vi "1.2.vi"() -> ()   [LabVIEW 2020]
panel:
  in  "Knob":dbl(knob) scale=0.0..10.0
  out "Meter":dbl(knob) scale=0.0..10.0
  out "Boolean 2":bool
  in  "Boolean":bool
  out "Numeric 2":i64
  in  "Numeric":i64
  out "String 2":string
  in  "String":string
  # "Tipo String"
  # "Tipo INT"
  # "Tipo Boolean"
  # "Tipo DBL"
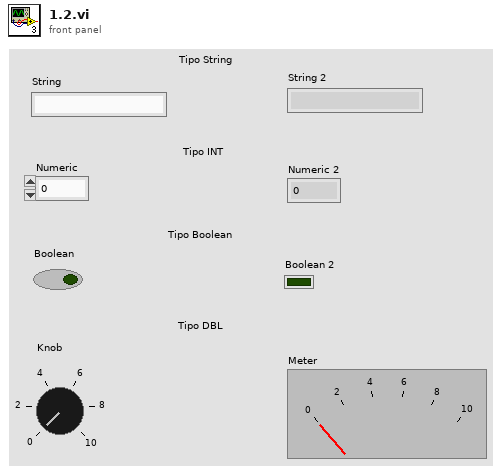
[diagram p1: front panel]
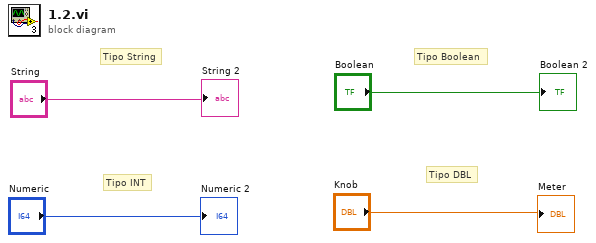
[diagram p0: block diagram]
diagram:
  # "Tipo DBL"
  # "Tipo Boolean"
  # "Tipo INT"
  # "Tipo String"
  "String 2" <- "String"
  "Numeric 2" <- "Numeric"
  "Boolean 2" <- "Boolean"
  "Meter" <- "Knob"
